vi "Read FPGA Ref.vi"(8 "error in (no error)":errorcluster, 11 "tCRD in":refnum<class "Open Path CRD.lvclass">) -> (0 "error out":errorcluster, 2 "FPGA Ref":T1, 3 "tCRD out":refnum<class "Open Path CRD.lvclass">)   [LabVIEW 2015, in "Open Path CRD.lvclass"]
uses:
  Open Path CRD.lvclass
  Open Path FPGA Ref.ctl
  Open Path CRD.lvclass/Open Path CRD.ctl
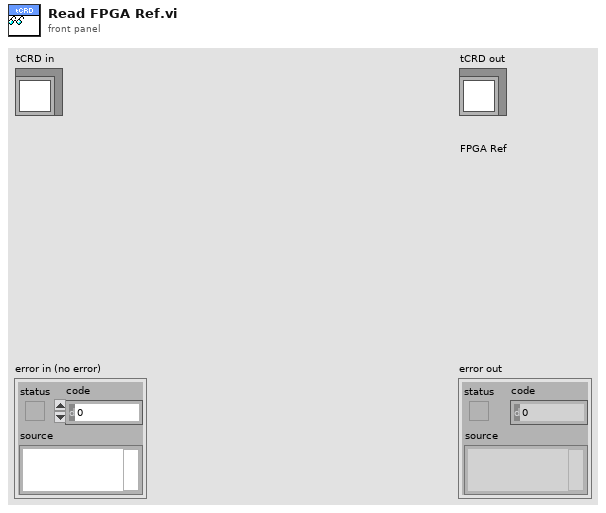
[diagram p1: front panel]
types:
  T1 = typedef "Open Path CRD.lvclass/Open Path FPGA Ref.ctl" = refnum<k20>
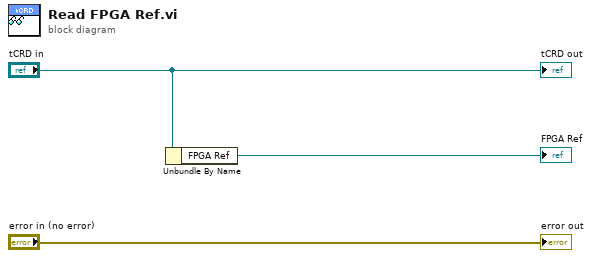
[diagram p0: block diagram]
diagram:
  n1 = Unbundle By Name("tCRD in") -> ("FPGA Ref"=→"FPGA Ref":T1)
  "error out" <- "error in (no error)"
  "tCRD out" <- "tCRD in"
